vi "PID-DruckRegler.vi"(0 "Sollwert":sgl, 1 "Regler EIN":bool=TRUE, 2 "Regler Interne Werte":sgl[](array[numeric]), 5 "Istwert":sgl, 7 "PID-Parameter":T2 {"Regler Toleranz -" format="%_2f"; "Regler Toleranz +" format="%_2f"; "D-Anteil" format="%_2f"; "I-Anteil" format="%_2f"; "P-Anteil" format="%_2f"}, 9 "output range":cluster{"output high":sgl, "output low":sgl}={"output high"=100.0, "output low"=-100.0} {"output low" format="%.2f"; "output high" format="%.2f"}, 11 "Dichtheitstest":bool=TRUE, 12 "Regler Toleranz verwenden?":bool=TRUE) -> (3 "Regler Interne Werte":T1, 4 "Interne Werte speichern":bool, 8 "Output":sgl)   [LabVIEW 2020, in "Regler.lvlib" / "Druckregler.lvlib"]
uses:
  Druckregler.lvlib
  Regler Interne Werte.ctl
  Regler Werte erzwingen.ctl
  <vilib>/addons/control/pid/pid.llb/PID Control Input Filter (DBL).vi
  <vilib>/addons/control/pid/NI_PID_pid.lvlib
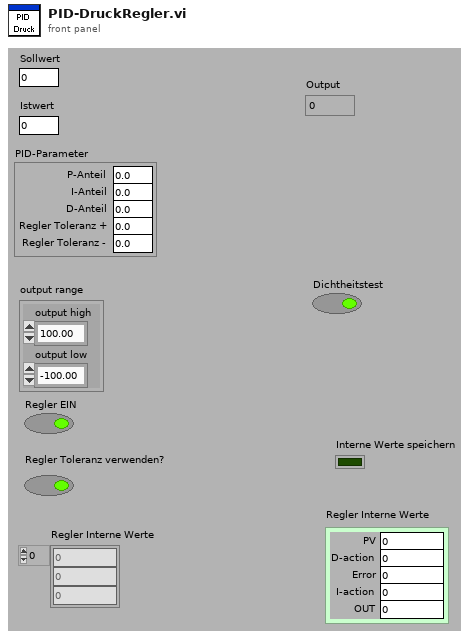
[diagram p1: front panel]
types:
  T1 = typedef "Regler.lvlib/Druckregler.lvlib/Regler Interne Werte.ctl" = cluster{"PV":sgl, "D-action":sgl, "Error":sgl, "I-action":sgl, "OUT":sgl}
  T2 = cluster{"P-Anteil":sgl, "I-Anteil":sgl, "D-Anteil":sgl, "Regler Toleranz +":sgl, "Regler Toleranz -":sgl}
  T3 = typedef "Regler.lvlib/Druckregler.lvlib/Regler Werte erzwingen.ctl" = enum16{"normal", "erzwingen"}
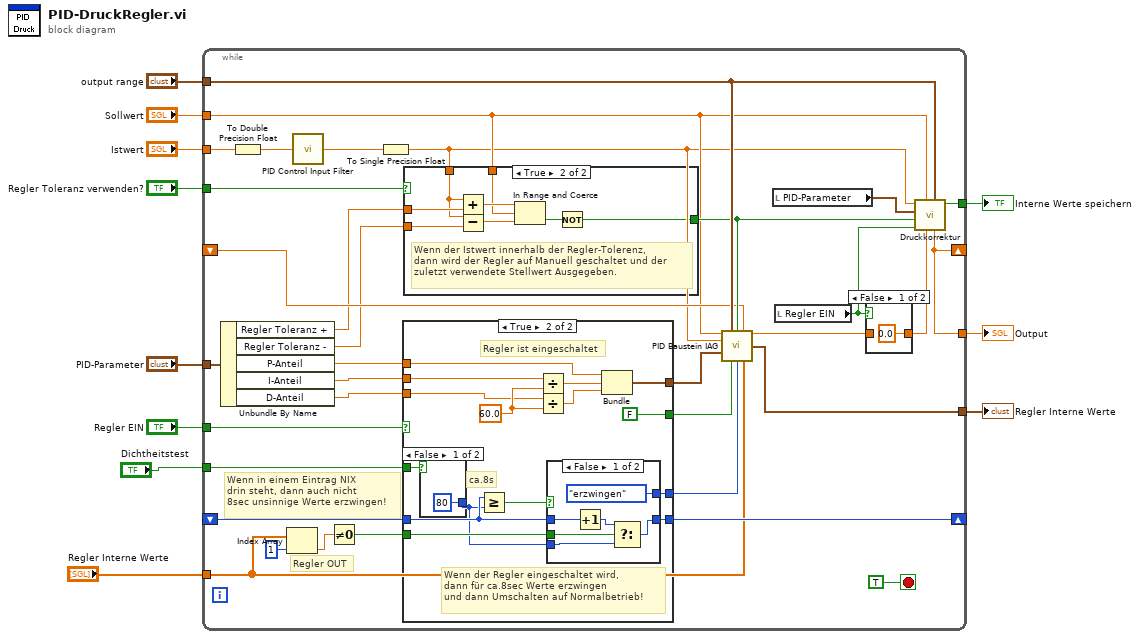
[diagram p0: block diagram]
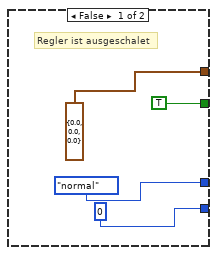
[diagram p2: hidden frame]
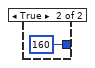
[diagram p3: hidden frame]
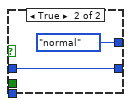
[diagram p4: hidden frame]
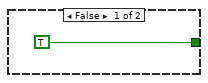
[diagram p5: hidden frame]
diagram:
  n1 = while {
    tunnel: "PID-Parameter" -> [w45]
    tunnel: "Regler EIN" -> [w41]
    tunnel: "Regler Toleranz verwenden?" -> [w37]
    tunnel: "output range" -> [w36]
    tunnel: [w21] -> w7
    tunnel: "Sollwert" -> [w16]
    tunnel: "Istwert" -> [w33]
    tunnel: [w28] -> w4
    tunnel: "Regler Interne Werte" -> [w19]
    shift-right: [w26] -> _
    shift-left: _ -> [w25]
    tunnel: [w23] -> w3
    shift-right: [w21] -> _
    shift-left: _ -> [w20]
    tunnel: "Dichtheitstest" -> [w12]
    stop <- TRUE stop-if-true
    # "Regler OUT"
    # "Wenn in einem Eintrag NIX\ndrin steht, dann auch nicht \n8sec unsinnige Werte erzwingen!"
    n2 = Unbundle By Name(w45) -> ("Regler Toleranz +"=w14:sgl, "Regler Toleranz -"=w13:sgl, "P-Anteil"=w44:sgl, "I-Anteil"=w43:sgl, "D-Anteil"=w42:sgl)
    n3 = To Double Precision Float(number=w33) -> (double precision float=w32:dbl)
    n4 = Index Array(array=w19, index=1 ("Index")) -> (element=w17:sgl)
    n5 = call-poly <vilib>:"PID Control Input Filter.vi"("input"=w32) -> ("output"=w31:dbl)  [unwired: 4 in]
    n6 = Not Equal To 0?(x=w17) -> (x != 0?=w22:bool)
    n7 = To Single Precision Float(number=w31) -> (single precision float=w15:sgl)
    n8 = case shown="True" w41 {
      tunnel: [cluster{"P-Anteil":sgl, sgl, sgl} {"P-Anteil"=0.0, 0.0, 0.0} w57] -> w40
      tunnel: w44 -> [_ w58]
      tunnel: w43 -> [_ w62]
      tunnel: w42 -> [_ w61]
      tunnel: [TRUE FALSE] -> w39
      tunnel: [u16 0 w56] -> w26
      tunnel: w25 -> [_ w55]
      tunnel: [Regler_Werte_erzwingen."normal" ("Regler erzwingen") w54] -> w24
      tunnel: w22 -> [_ w53]
      tunnel: w12 -> [_ w51]
      frame False {
        # "Regler ist ausgeschalet"
      }
      frame True {
        w63 = sgl 60.0 ("y")
        # "Wenn der Regler eingeschaltet wird, \ndann für ca.8sec Werte erzwingen \nund dann Umschalten auf Normalbetrieb!"
        # "ca.8s"
        # "Regler ist eingeschaltet"
        n9 = case shown="False" w51 {
          tunnel: [u16 80 ("y") u16 160 ("y")] -> w50
          frame False {
          }
          frame True {
          }
        }
        n10 = Greater Or Equal?(x=w55, y=w50) -> (x >= y?=w52:bool)
        n11 = Divide(x=w62, y=w63) -> (x/y=w60:sgl)
        n12 = Divide(x=w61, y=w63) -> (x/y=w59:sgl)
        n13 = case shown="False" w52 {
          tunnel: w55 -> [w72 w74]
          tunnel: [w68 w74] -> w56
          tunnel: [Regler_Werte_erzwingen."erzwingen" ("Regler erzwingen") Regler_Werte_erzwingen."normal" ("Regler erzwingen")] -> w54
          tunnel: w53 -> [w70 _]
          tunnel: w50 -> [w67 _]
          frame False {
            n14 = Increment(x=w72) -> (x+1=w69:u16)
            n15 = Select(t=w69, s=w70, f=w67) -> (s? t:f=w68:u16)
          }
          frame True {
          }
        }
        n16 = Bundle("P-Anteil"=w58, w60, w59) -> (w57:cluster{"P-Anteil":sgl, sgl, sgl})  [unwired: 1 in]
      }
    }
    n17 = case shown="True" w37 {
      tunnel: [TRUE w82] -> w35
      tunnel: w15 -> [_ w77]
      tunnel: w14 -> [_ w81]
      tunnel: w13 -> [_ w80]
      tunnel: w16 -> [_ w76]
      frame False {
      }
      frame True {
        # "Wenn der Istwert innerhalb der Regler-Tolerenz,\ndann wird der Regler auf Manuell geschaltet und der \nzuletzt verwendete Stellwert Ausgegeben."
        n18 = Add(x=w77, y=w81) -> (x+y=w79:sgl)
        n19 = Subtract(x=w77, y=w80) -> (x-y=w78:sgl)
        n20 = In Range and Coerce(upper limit=w79, x=w76, lower limit=w78) -> (In Range?=w83:bool)  [unwired: 1 out]
        n21 = Not(x=w83) -> (.not. x?=w82:bool)
      }
    }
    n22 = call "PID Baustein IAG.vi"("setpoint"=w16, "output range"=w36, "auto? (T)"=w35, "manual control"=w20, "process variable"=w15, "PID gains"=w40, "reinitialize? (F)"=w39, "Regler erzwingen"=w24, "Regler Interne Werte"=w19) -> ("output"=w38:sgl, "Regler Werte"=w28:T1)  [unwired: 4 in, 1 out]
    n23 = local read "PID-Parameter"() -> (w30:T2)
    n24 = local read "Regler EIN"() -> (w29:bool)
    n25 = case shown="False" w29 {
      tunnel: [sgl 0.0 w85] -> w34
      tunnel: w38 -> [_ w85]
      frame False {
      }
      frame True {
      }
    }
    n26 = call "Druckkorrektur.vi"("output range"=w36, "Output"=w34, "Sollwert"=w16, "Regler EIN"=w29, "Auto?"=w35, "PID-Parameter"=w30, "Istwert"=w15) -> ("Interne Werte speichern"=w23:bool, "Output"=w21:sgl)  [unwired: 3 in]
  }
  "Output" <- w7
  "Regler Interne Werte" <- w4
  "Interne Werte speichern" <- w3
